vi "Sub_Slope.vi"(1 "X":dbl[](array[numeric]), 2 "Y":dbl[](array[numeric])) -> (0 "slope":dbl)   [LabVIEW 2014]
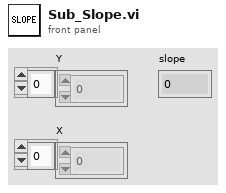
[diagram p1: front panel]
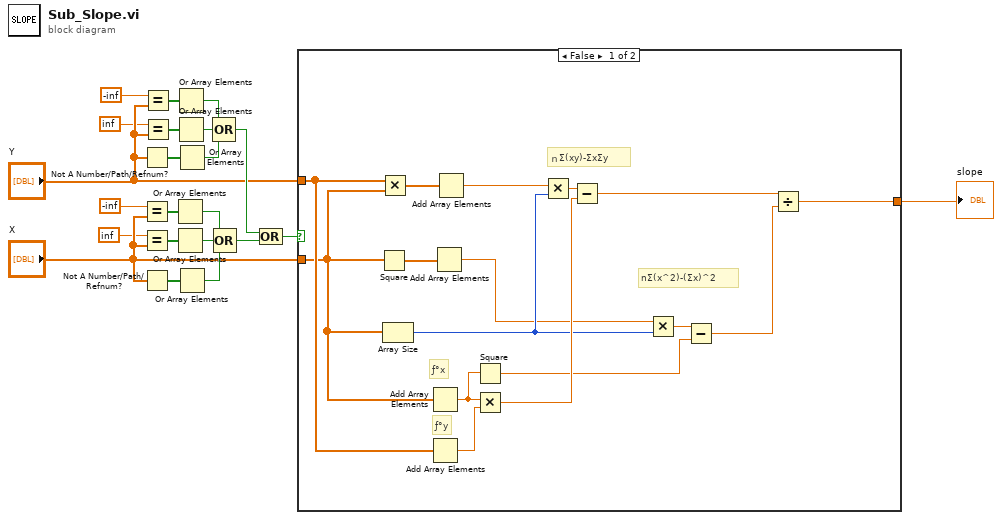
[diagram p0: block diagram]
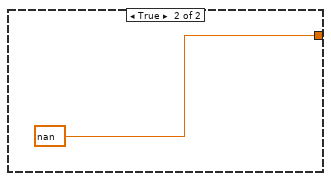
[diagram p2: hidden frame]
diagram:
  n1 = Not A Number/Path/Refnum?(number/path/refnum="Y") -> (NaN/Path/Refnum?=w2:bool[])
  n2 = Equal?(x=-inf, y="X") -> (x = y?=w13:bool[])
  n3 = Equal?(x=inf, y="X") -> (x = y?=w14:bool[])
  n4 = Not A Number/Path/Refnum?(number/path/refnum="X") -> (NaN/Path/Refnum?=w3:bool[])
  n5 = Equal?(x=-inf, y="Y") -> (x = y?=w9:bool[])
  n6 = Equal?(x=inf, y="Y") -> (x = y?=w8:bool[])
  n7 = Or Array Elements(Boolean array=w13) -> (logical OR=w19:bool)
  n8 = Or Array Elements(Boolean array=w14) -> (logical OR=w18:bool)
  n9 = Or Array Elements(Boolean array=w9) -> (logical OR=w11:bool)
  n10 = Or Array Elements(Boolean array=w8) -> (logical OR=w10:bool)
  n11 = Or Array Elements(Boolean array=w2) -> (logical OR=w12:bool)
  n12 = Or Array Elements(Boolean array=w3) -> (logical OR=w20:bool)
  n13 = Compound Arithmetic op=OR(w11, w10, w12) -> (w22:bool)
  n14 = Compound Arithmetic op=OR(w19, w18, w20) -> (w21:bool)
  n15 = Compound Arithmetic op=OR(w22, w21) -> (w4:bool)
  n16 = case shown="FALSE" w4 {
    tunnel: [w23 nan ("slope")] -> w1
    tunnel: "Y" -> [w36 _]
    tunnel: "X" -> [w27 _]
    frame False {
      # "nΣ(x^2)-(Σx)^2"
      # "ƒ°x"
      # "ƒ°y"
      # "ｎΣ(xy)-ΣxΣy"
      n17 = Square(x=w27) -> (x^2=w29:dbl[])
      n18 = Multiply(x=w36, y=w27) -> (x*y=w38:dbl[])
      n19 = Array Size(array=w27) -> (size(s)=w32:i32)
      n20 = Add Array Elements(numeric array=w27) -> (sum=w31:dbl)
      n21 = Add Array Elements(numeric array=w36) -> (sum=w35:dbl)
      n22 = Add Array Elements(numeric array=w29) -> (sum=w28:dbl)
      n23 = Add Array Elements(numeric array=w38) -> (sum=w37:dbl)
      n24 = Square(x=w31) -> (x^2=w26:dbl)
      n25 = Multiply(x=w31, y=w35) -> (x*y=w33:dbl)
      n26 = Multiply(x=w37, y=w32) -> (x*y=w34:dbl)
      n27 = Subtract(x=w34, y=w33) -> (x-y=w25:dbl)
      n28 = Multiply(x=w28, y=w32) -> (x*y=w30:dbl)
      n29 = Subtract(x=w30, y=w26) -> (x-y=w24:dbl)
      n30 = Divide(x=w25, y=w24) -> (x/y=w23:dbl)
    }
    frame True {
    }
  }
  "slope" <- w1
